vi "fftw__memcpy_to_cplx_poly.vi"   [LabVIEW 2020, in "FFTWDLL.lvlib"]
doc: "Copy FFTW cplx aligned array to LV cplx array."
uses:
  FFTWDLL.lvlib
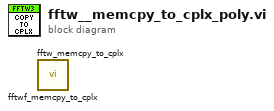
[diagram p0: block diagram]
diagram:
  n1 = call "fftwf_memcpy_to_cplx.vi"() -> ()  [unwired: 9 in, 3 out]
  n2 = call "fftw_memcpy_to_cplx.vi"() -> ()  [unwired: 9 in, 3 out]
